vi "Latihan 5 (Flat Sequence).vi"() -> ()   [LabVIEW 2021]
panel:
  out "LED 3":bool
  out "LED 2":bool
  out "LED 1":bool
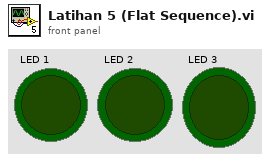
[diagram p1: front panel]
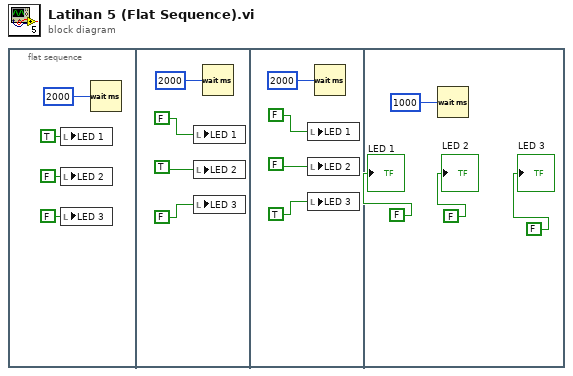
[diagram p0: block diagram]
diagram:
  n1 = flat-sequence {
    frame #0 {
      n2 = local write "LED 1"(TRUE) -> ()
      n3 = local write "LED 2"(FALSE) -> ()
      n4 = local write "LED 3"(FALSE) -> ()
      n5 = Wait (ms)(milliseconds to wait=u32 2000) -> ()  [unwired: 1 out]
    }
    frame #1 {
      n6 = local write "LED 1"(FALSE) -> ()
      n7 = local write "LED 2"(TRUE) -> ()
      n8 = local write "LED 3"(FALSE) -> ()
      n9 = Wait (ms)(milliseconds to wait=u32 2000) -> ()  [unwired: 1 out]
    }
    frame #2 {
      n10 = local write "LED 1"(FALSE) -> ()
      n11 = local write "LED 2"(FALSE) -> ()
      n12 = local write "LED 3"(TRUE) -> ()
      n13 = Wait (ms)(milliseconds to wait=u32 2000) -> ()  [unwired: 1 out]
    }
    frame #3 {
      n14 = Wait (ms)(milliseconds to wait=u32 1000) -> ()  [unwired: 1 out]
      "LED 3" <- FALSE
      "LED 2" <- FALSE
      "LED 1" <- FALSE
    }
  }
